vi "DSF.Engine.Memory.BufferPool.Allocate.vi"(8 "error in (no error)":errorcluster, 10 "size per buffer":u64 format="%d bytes", 11 "number of buffers":u32 format="%d buffers") -> (0 "error out":errorcluster, 3 "BufferPool":refnum<class "DSF.Engine.Memory.BufferPool.lvclass">)   [LabVIEW 2016, in "DSF.Engine.lvlib" / "DSF.Engine.Memory.BufferPool.lvclass"]
uses:
  DSF.Engine.Memory.BufferPool.lvclass
  DSF.Engine.Memory.BufferPool.lvclass/DSF.Engine.Memory.BufferPool.ctl
  Buffer/DSF.Engine.Memory.Buffer.lvclass
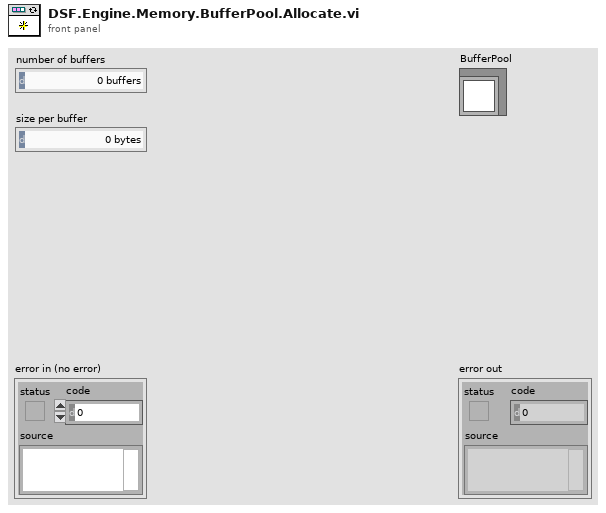
[diagram p1: front panel]
types:
  T1 = cluster{"read mode":enum16{"polling", "blocking"}, "write mode":enum16{"polling", "blocking"}}
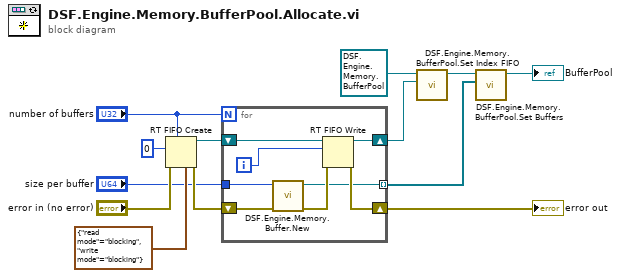
[diagram p0: block diagram]
diagram:
  n1 = RT FIFO Create(1:0, 3:"error in (no error)", 4:"number of buffers", 7:T1 {"read mode"=enum."blocking", "write mode"=enum."blocking"} ("r/w modes (polling,polling)")) -> (8:w11:refnum<k33>, 11:w9:errorcluster)  [unwired: 4 in, 1 out]
  n2 = for {
    N: "number of buffers" -> [_]
    tunnel: "size per buffer" -> [w21]
    shift-right: [w17] -> w4
    shift-left: w9 -> [w20]
    shift-right: [w18] -> w3
    shift-left: w11 -> [w19]
    tunnel: [w15] -> w5 mode=indexing
    i -> [w14]
    n3 = call "DSF.Engine.Memory.Buffer.New.vi"("error in (no error)"=w20, "size"=w21) -> ("error out"=w16:errorcluster, "Buffer out"=w15:refnum<class "DSF.Engine.Memory.Buffer.lvclass">)  [unwired: 8 in]
    n4 = RT FIFO Write(0:w19, 1:w14, 3:w16) -> (8:w18:refnum<k33>, 11:w17:errorcluster)  [unwired: 2 in, 2 out]
  }
  "error out" <- w4
  n5 = call "DSF.Engine.Memory.BufferPool.Set Index FIFO.vi"("Index FIFO"=w3, "BufferPool in"=refnum<class "DSF.Engine.Memory.BufferPool.lvclass"> refnum ("BufferPool")) -> ("BufferPool out"=w7:refnum<class "DSF.Engine.Memory.BufferPool.lvclass">)  [unwired: 8 in, 1 out]
  n6 = call "DSF.Engine.Memory.BufferPool.Set Buffers.vi"("Buffers"=w5, "BufferPool in"=w7) -> ("BufferPool out"=→"BufferPool":refnum<class "DSF.Engine.Memory.BufferPool.lvclass">)  [unwired: 8 in, 1 out]
